vi "Return Actual Points.vi"(8 "error in (no error)":errorcluster, 9 "Total Points (2000)":i32=2000, 10 "Offset (0)":i32, 11 "Number of Samples (1000)":i32=1000) -> (0 "error out":errorcluster, 3 "Actual Points":i32)   [LabVIEW 2020, in "Agilent 90000 Series.lvlib"]
doc: "Returns the actual points by the number of samples, offset and total points in the instrument memory buffer."
uses:
  Agilent 90000 Series.lvlib
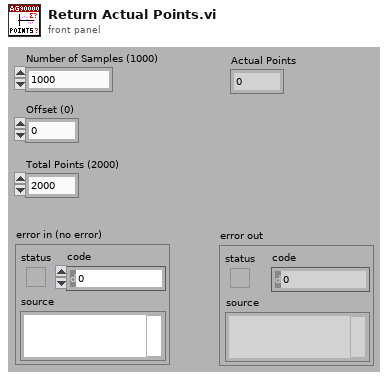
[diagram p1: front panel]
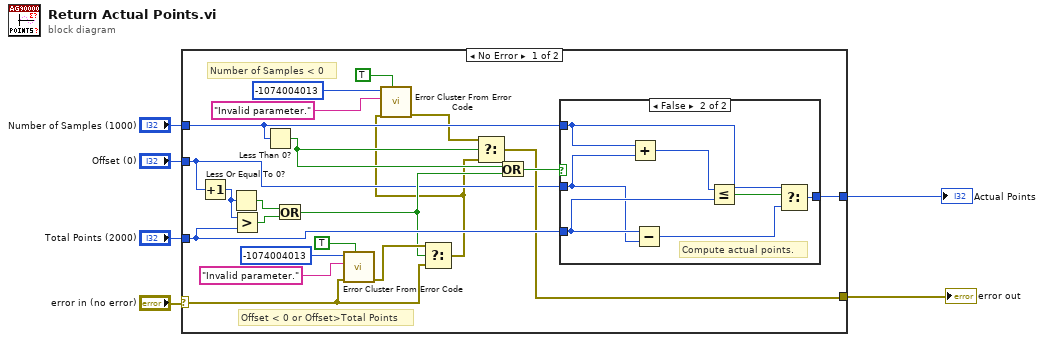
[diagram p0: block diagram]
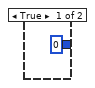
[diagram p2: hidden frame]
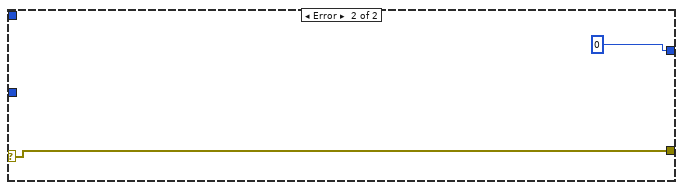
[diagram p3: hidden frame]
diagram:
  n1 = case shown="No Error" "error in (no error)" {
    selector: "error in (no error)" -> [w8 w37]
    tunnel: "Total Points (2000)" -> [w26 _]
    tunnel: "Offset (0)" -> [w10 _]
    tunnel: "Number of Samples (1000)" -> [w19 _]
    tunnel: [w27 0 ("Number of Samples")] -> w3
    tunnel: [w11 w37] -> w1
    frame No Error {
      # "Number of Samples < 0"
      # "Offset < 0 or Offset>Total Points"
      n2 = Increment(x=w10) -> (x+1=w9:i32)
      n3 = Less Or Equal To 0?(x=w9) -> (x <= 0?=w25:bool)
      n4 = Greater?(x=w9, y=w26) -> (0:w24:bool)
      n5 = Less Than 0?(x=w19) -> (x < 0?=w14:bool)
      n6 = Or(x=w25, y=w24) -> (x .or. y?=w13:bool)
      n7 = call <vilib>:"Error Cluster From Error Code.vi"("show call chain? (False)"=TRUE, "error in (no error)"=w8, "error message (\"\")"="Invalid parameter." ("error message (\"\")"), "error code (0)"=-1074004013) -> ("error out"=w20:errorcluster)  [unwired: 5 in]
      n8 = Select(t=w20, s=w13, f=w8) -> (s? t:f=w7:errorcluster)
      n9 = call <vilib>:"Error Cluster From Error Code.vi"("show call chain? (False)"=TRUE, "error in (no error)"=w7, "error message (\"\")"="Invalid parameter." ("error message (\"\")"), "error code (0)"=-1074004013) -> ("error out"=w15:errorcluster)  [unwired: 5 in]
      n10 = Select(t=w15, s=w14, f=w7) -> (s? t:f=w11:errorcluster)
      n11 = Or(x=w14, y=w13) -> (x .or. y?=w12:bool)
      n12 = case shown="False" w12 {
        tunnel: [0 ("Number of Samples") w35] -> w27
        tunnel: w10 -> [_ w29]
        tunnel: w26 -> [_ w32]
        tunnel: w19 -> [_ w31]
        frame True {
        }
        frame False {
          # "Compute actual points."
          n13 = Add(x=w31, y=w29) -> (x+y=w30:i32)
          n14 = Subtract(x=w32, y=w29) -> (x-y=w33:i32)
          n15 = Less Or Equal?(x=w30, y=w32) -> (x <= y?=w34:bool)
          n16 = Select(t=w31, s=w34, f=w33) -> (s? t:f=w35:i32)
        }
      }
    }
    frame Error {
    }
  }
  "Actual Points" <- w3
  "error out" <- w1
